vi "mxwScript_Cmnd2Str_setObjectValue.vi"(8 "error in (no error)":errorcluster, 11 "data":variant) -> (0 "error out":errorcluster, 3 "outputString":string)   [LabVIEW 2020]
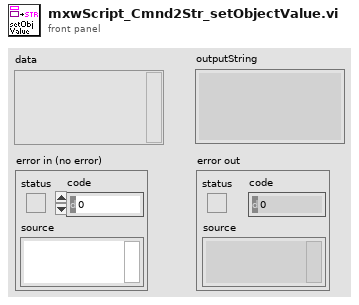
[diagram p1: front panel]
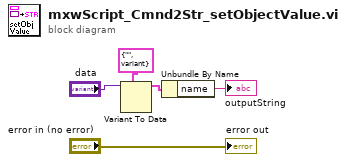
[diagram p0: block diagram]
diagram:
  n1 = Variant To Data(type=cluster{"name":string, "value":variant} {"name"="", "value"=variant} ("parameter"), Variant="data") -> (data=w2:cluster{"name":string, "value":variant})  [unwired: 1 in, 1 out]
  n2 = Unbundle By Name(w2) -> ("name"=→"outputString":string)
  "error out" <- "error in (no error)"
